vi "ejercicio1.vi"() -> ()   [LabVIEW 2020]
panel:
  out "Area":dbl
  in  "Base":dbl
  in  "Altura":dbl
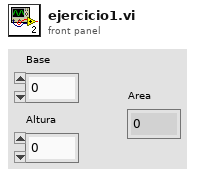
[diagram p1: front panel]
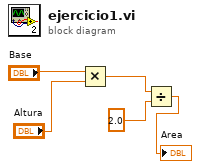
[diagram p0: block diagram]
diagram:
  n1 = Multiply(x="Base", y="Altura") -> (x*y=w1:dbl)
  n2 = Divide(x=w1, y=2.0) -> (x/y=→"Area":dbl)
